vi "TestTreeToRepo.vi"() -> (2 "summary":T1[](array[typedef]))   [LabVIEW 2013]
uses:
  Trunk/vi.lib/CEF_TreeControl/Node/Summary.ctl
  Controls/IDs.ctl
  Trunk/ProjectTemplates/Source/Configuration Editor Framework/Classes/cRIO/cRIO.lvclass
  Trunk/ProjectTemplates/Source/Configuration Editor Framework/Classes/Group/Group.lvclass
  Trunk/ProjectTemplates/Source/Configuration Editor Framework/Classes/Voltage/Voltage.lvclass
  Trunk/ProjectTemplates/Source/Configuration Editor Framework/Classes/cRIO Repo/cRIORepo.lvclass
  Trunk/vi.lib/CEF_TreeControl/Node/NISE_CEF_Node.lvclass
  Trunk/vi.lib/CEF_TreeControl/NISE_CEF_TreeControl.lvlib
panel:
  out "summary 4":T1[](array[typedef])
  out "summary 3":T1[](array[typedef])
  out "Ids 4":T2
  out "Ids 3":T2
  out "Ids 2":T2
  out "Ids":T2
  out "summary 2":T1[](array[typedef])
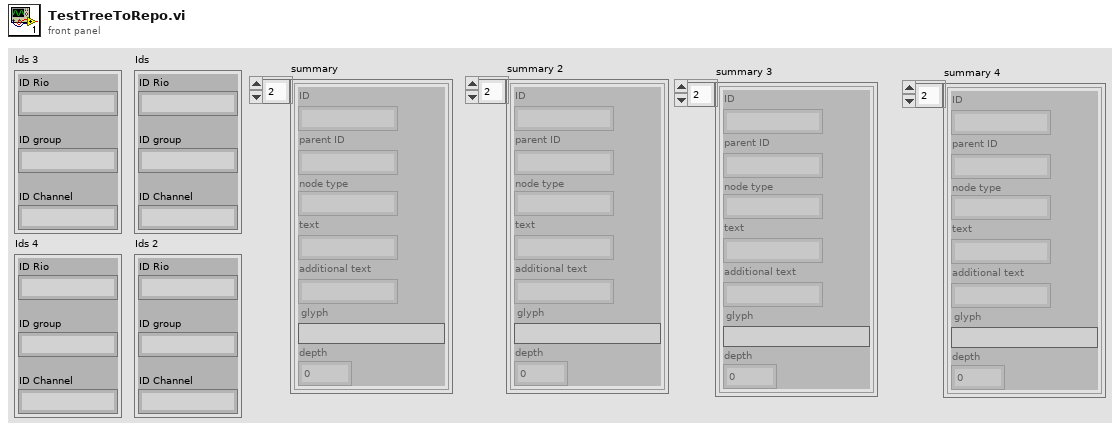
[diagram p1: front panel]
types:
  T1 = typedef "NISE_CEF_Node.lvclass/Summary.ctl" = cluster{"ID":string, "parent ID":string, "node type":string, "text":string, "additional text":string, "glyph":string, "depth":i32}
  T2 = typedef "IDs.ctl" = cluster{"ID Channel":string, "ID Rio":string, "ID group":string}
  T3 = typedef "NISE_CEF_Node.lvclass/NodeRef.ctl" = refnum<data-value>
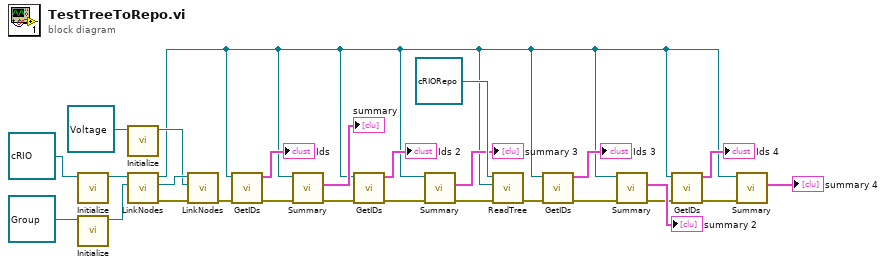
[diagram p0: block diagram]
diagram:
  n1 = call-dynamic "Initialize.vi"("cRIO in"=refnum<class "cRIO.lvclass"> refnum ("cRIO.lvclass")) -> ("data value reference"=w24:T3)  [unwired: 8 in, 2 out]
  n2 = call-dynamic "Initialize.vi"("group in"=refnum<class "Group.lvclass"> refnum ("Group.lvclass")) -> ("data value reference"=w23:T3)  [unwired: 8 in, 2 out]
  n3 = call-dynamic "Initialize.vi"("voltage in"=refnum<class "Voltage.lvclass"> refnum ("Voltage.lvclass")) -> ("data value reference"=w21:T3)  [unwired: 8 in, 2 out]
  n4 = call "LinkNodes.vi"("child in"=w23, "parent in"=w24) -> ("error out"=w18:errorcluster, "child out"=w22:T3, "parent out"=w3:T3)  [unwired: 7 in]
  n5 = call "LinkNodes.vi"("error in"=w18, "child in"=w21, "parent in"=w22) -> ("error out"=w17:errorcluster)  [unwired: 6 in, 2 out]
  n6 = call "GetIDs.vi"("error in"=w17, "data value reference in"=w3) -> ("error out"=w16:errorcluster, "IDs"=→"Ids":T2)  [unwired: 6 in, 2 out]
  n7 = call "Summary.vi"("error in"=w16, "node self ref"=w3) -> ("error out"=w14:errorcluster, "summary"=→"summary":T1[])  [unwired: 8 in]
  n8 = call "GetIDs.vi"("error in"=w14, "data value reference in"=w3) -> ("error out"=w9:errorcluster, "IDs"=→"Ids 2":T2)  [unwired: 6 in, 2 out]
  n9 = call "Summary.vi"("error in"=w9, "node self ref"=w3) -> ("error out"=w7:errorcluster, "summary"=→"summary 3":T1[])  [unwired: 8 in]
  n10 = call-dynamic "ReadTree.vi"("error in"=w7, "root"=w3, "cRIO repo in"=refnum<class "cRIORepo.lvclass"> refnum ("cRIORepo.lvclass")) -> ("error out"=w12:errorcluster)  [unwired: 7 in, 1 out]
  n11 = call "GetIDs.vi"("error in"=w12, "data value reference in"=w3) -> ("error out"=w6:errorcluster, "IDs"=→"Ids 3":T2)  [unwired: 6 in, 2 out]
  n12 = call "Summary.vi"("error in"=w6, "node self ref"=w3) -> ("error out"=w4:errorcluster, "summary"=→"summary 2":T1[])  [unwired: 8 in]
  n13 = call "GetIDs.vi"("error in"=w4, "data value reference in"=w3) -> ("error out"=w1:errorcluster, "IDs"=→"Ids 4":T2)  [unwired: 6 in, 2 out]
  n14 = call "Summary.vi"("error in"=w1, "node self ref"=w3) -> ("summary"=→"summary 4":T1[])  [unwired: 8 in, 1 out]
